vi "Select_GEA2_GEA3.vi"(0 "session in":refnum<k35>, 2 "GEA2 or GEA3":T1, 7 "Board":u8, 11 "error in (no error)":errorcluster) -> (4 "session out":refnum<k35>, 8 "isGEA3?":bool, 15 "error out":errorcluster)   [LabVIEW 2021]
uses:
  Controles/Select_GEA2_OR_GEA3.ctl
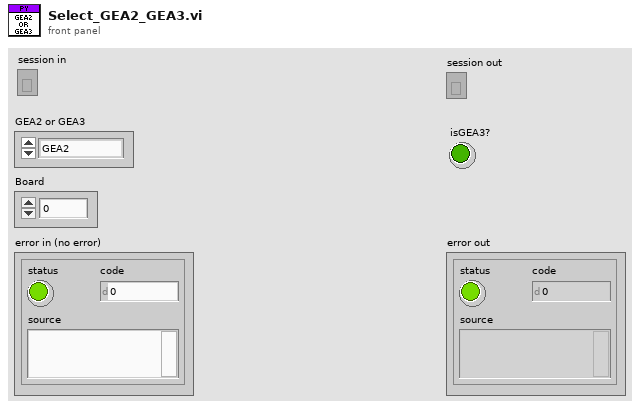
[diagram p1: front panel]
types:
  T1 = typedef "Select_GEA2_OR_GEA3.ctl" = enum16{"GEA2", "GEA3"}
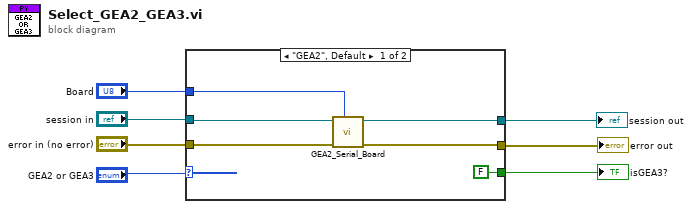
[diagram p0: block diagram]
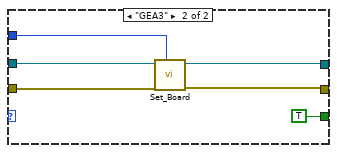
[diagram p2: hidden frame]
diagram:
  n1 = case shown="\"GEA2\", Default" "GEA2 or GEA3" {
    tunnel: "session in" -> [w13 w19]
    tunnel: "error in (no error)" -> [w12 w18]
    tunnel: [w11 w17] -> w4
    tunnel: [w10 w16] -> w3
    tunnel: "Board" -> [w8 w15]
    tunnel: [FALSE TRUE] -> w1
    frame "GEA2", Default {
      n2 = call "GEA2_Serial_Board.vi"("Board"=w8, "error in (no error)"=w12, "session in"=w13) -> ("error out"=w10:errorcluster, "session out"=w11:refnum<k35>)  [unwired: 7 in]
    }
    frame "GEA3" {
      n3 = call "Set_Board.vi"("Board"=w15, "error in (no error)"=w18, "session in"=w19) -> ("error out"=w16:errorcluster, "session out"=w17:refnum<k35>)  [unwired: 7 in]
    }
  }
  "session out" <- w4
  "error out" <- w3
  "isGEA3?" <- w1
